vi "defects database show.vi"() -> ()   [LabVIEW 2019]
uses:
  database.lvlib
panel:
  out "error out":errorcluster
  in  "Close Square":bool
  in  "Refresh Button":bool
  out "DEFECTS  TABLE":string[][](table)
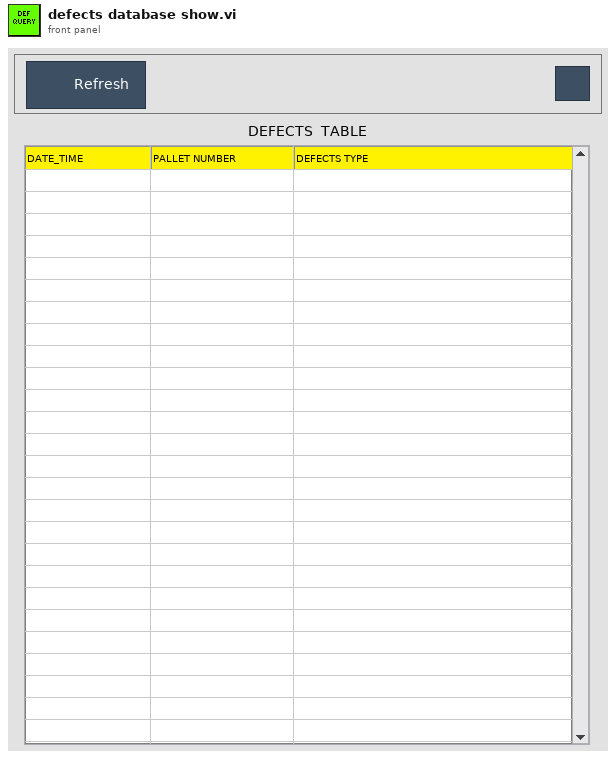
[diagram p1: front panel]
types:
  T1 = cluster{"plt number dis":i16, "Table Name":string, "Database Name":string, "DB days to save":i16, "IP #":string, "Img Path":path, "Port":u16, "time out":u16, "madule path":path, "IP # speed":string, "counting device":enum16{"Sensors", "Line Speed", "Sensors&Speed"}}
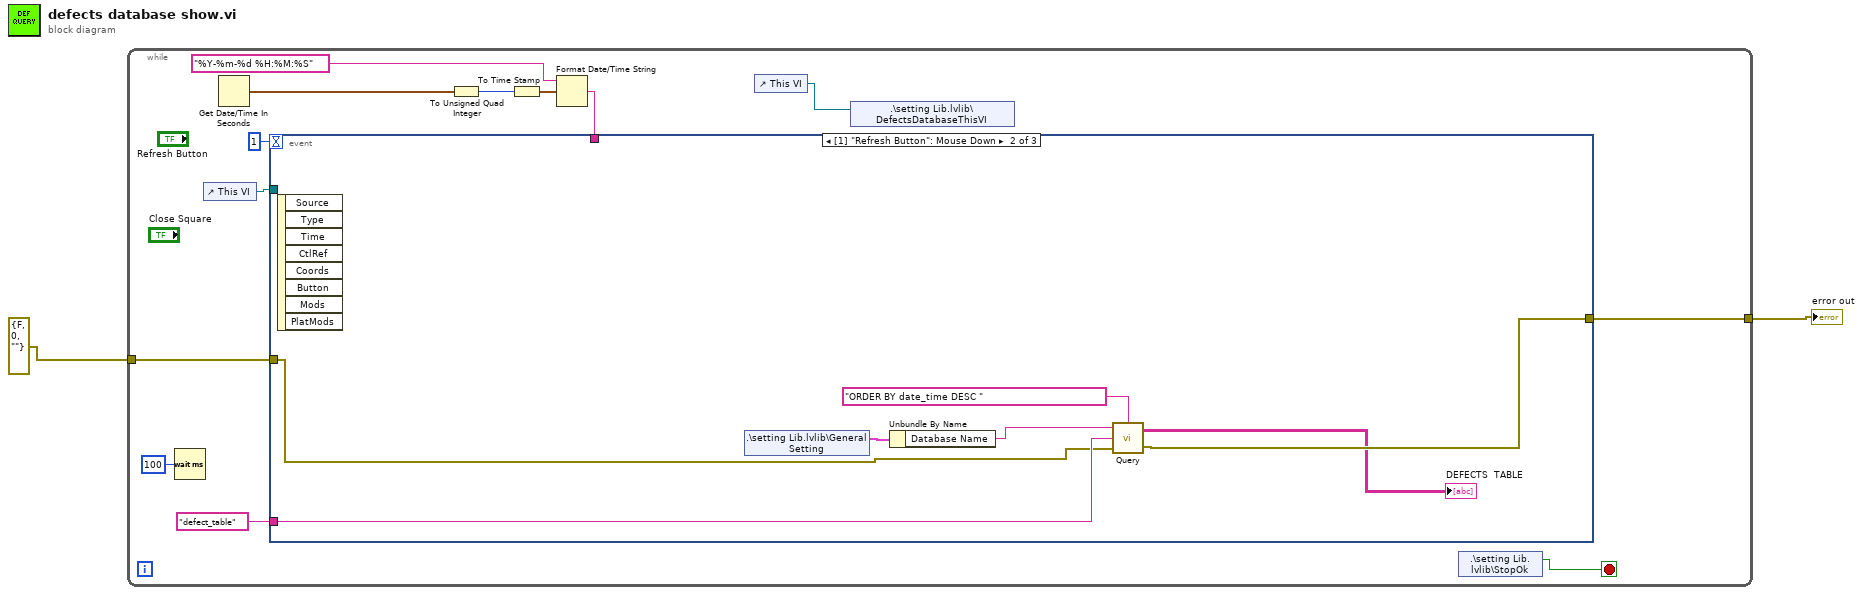
[diagram p0: block diagram]
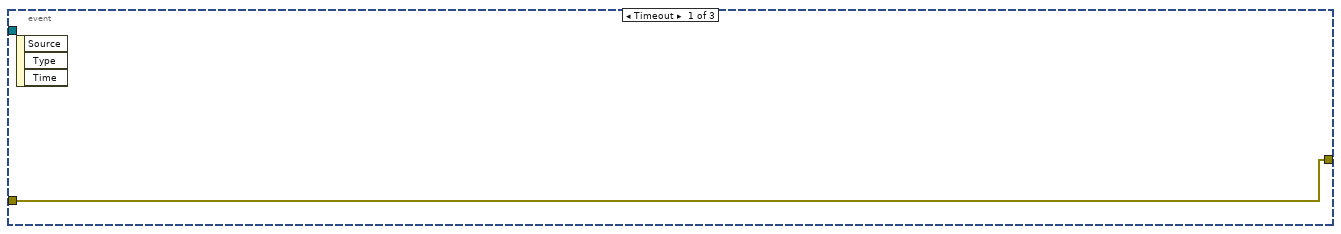
[diagram p2: hidden frame]
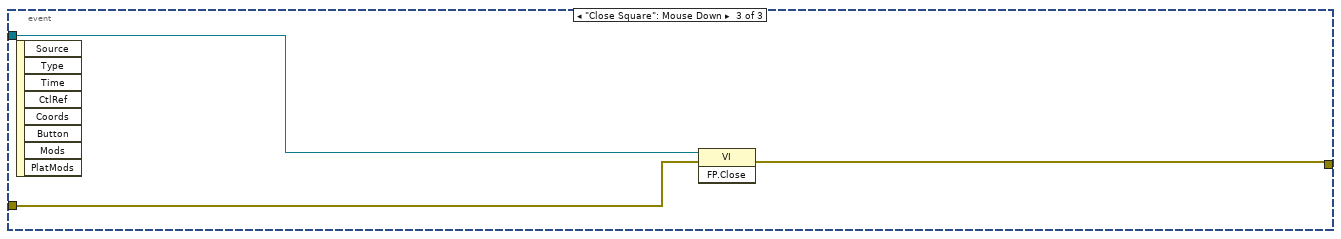
[diagram p3: hidden frame]
diagram:
  n1 = while {
    tunnel: errorcluster {"status"=FALSE, "code"=0, "source"=""} ("error in (no error)") -> [w5]
    tunnel: [w4] -> w1
    stop <- w6 stop-if-true
    n2 = Wait (ms)(milliseconds to wait=u32 100) -> ()  [unwired: 1 out]
    n3 = control-ref of="This VI"() -> (w7:refnum<vi>)
    n4 = Get Date/Time In Seconds() -> (seconds since 1Jan1904=w10:timestamp)
    n5 = To Unsigned Quad Integer(1:w10) -> (0:w11:u64)
    n6 = To Time Stamp(1:w11) -> (0:w12:timestamp)
    n7 = Format Date/Time String(time format string (%c)="%Y-%m-%d %H:%M:%S", seconds (now)=w12) -> (date/time string=w9:string)  [unwired: 1 in]
    n8 = event shown="[1] \"Refresh Button\": Mouse Down" {
      selector: _ -> [_ _ _]
      dyn-events: _ -> [_ _ _]
      timeout: 1 -> [_ _ _]
      tunnel: "defect_table" ("table") -> [_ w23 _]
      tunnel: w9 -> [_ _ _]
      tunnel: w5 -> [w16 w20 w26]
      tunnel: w7 -> [_ _ w25]
      tunnel: [w16 w19 w24] -> w4
      event Timeout {
        n9 = event-data() -> ()  [unwired: 1 in, 3 out]
      }
      event "Refresh Button": Mouse Down {
        n10 = event-data() -> ()  [unwired: 1 in, 8 out]
        n11 = shared-variable ".\\setting Lib.lvlib\\General Setting"() -> (w22:T1)  [unwired: 1 in, 1 out]
        n12 = Unbundle By Name(w22) -> ("Database Name"=w21:string)
        n13 = call "Query.vi"("Condition"="ORDER BY date_time DESC ", "Error in"=w20, "Table Name"=w23, "Connection Name"=w21) -> ("Error out"=w19:errorcluster, "data"=→"DEFECTS  TABLE":string[][])
      }
      event "Close Square": Mouse Down {
        n14 = event-data() -> ()  [unwired: 1 in, 8 out]
        n15 = invoke class="VI" method="FP.Close"(reference=w25, error in=w26) -> (error out=w24:errorcluster)  [unwired: 1 in, 2 out]
      }
    }
    n16 = control-ref of="This VI"() -> (w13:refnum<vi>)
    n17 = shared-variable ".\\setting Lib.lvlib\\DefectsDatabaseThisVI"(w13) -> ()  [unwired: 1 in, 1 out]
    n18 = shared-variable ".\\setting Lib.lvlib\\StopOk"() -> (w6:bool)  [unwired: 1 in, 1 out]
  }
  "error out" <- w1
